vi "Acquire_wp_nodt.vi"(1 "Command FIFO":refnum<k21>, 2 "Circular Buffer Mem":refnum<k21>, 3 "circular buffer length":u32=300, 5 "FPGA I/O In":refnum<k21>="IO Module\\AI A0", 6 "Timing FIFO":refnum<k21>, 7 "channel on/off":bool, 9 "Trigger":i16=1500, 11 "Samples to Acquire":u32=95, 12 "Is Test Pulse?":bool, 13 "# of pretrigger":u32=15, 14 "timing":u64) -> ()   [LabVIEW 2012]
uses:
  <vilib>/rvi/eio/common/nirviEmuTemplateMethod_errors.vi
  <vilib>/rvi/DataTransferAndStorage/Container/Common/niFpgaContainerExecOnDevCompGetState.vi
  <vilib>/rvi/Emulation/niFpgaSctlEmulationGetInTimedLoop.vi
  <vilib>/rvi/DataTransferAndStorage/Container/Common/niFpgaContainerGetUniqueNameForEmu.vi
  <vilib>/rvi/FIFO/Fifo_Resource/nirvififoEmulationSetSize.vi
  <vilib>/rvi/errors/niFpgaSetErrorForExecOnDevCompSimple.vi
  <vilib>/rvi/eio/common/nirviEmuReportErrorAndStop.vi
  <vilib>/rvi/Emulation/niFpgaSctlEmulationFifoFullMgr.vi
  <vilib>/rvi/Emulation/niFpgaSctlEmulationResourceMgr.vi
  <vilib>/rvi/interface/RandomDataEmulation/nirviRandomDataFPGAFIFO.vi
  <vilib>/rvi/interface/RandomDataEmulation/niFpgaRandomDataHandleErrors.vi
  <vilib>/eio/EIONode/EIONode.xnode
  <vilib>/rvi/DataTransferAndStorage/Container/XNode/niFpgaContainer.xnode
  <vilib>/rvi/FIFO/Fifo_Resource/niFpgaFifoEmulationRefIn.vi
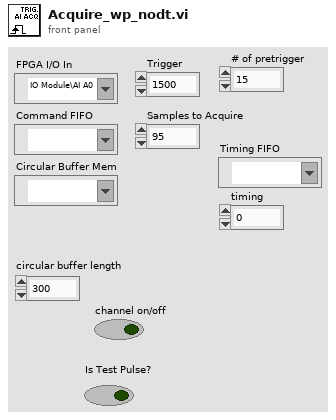
[diagram p1: front panel]
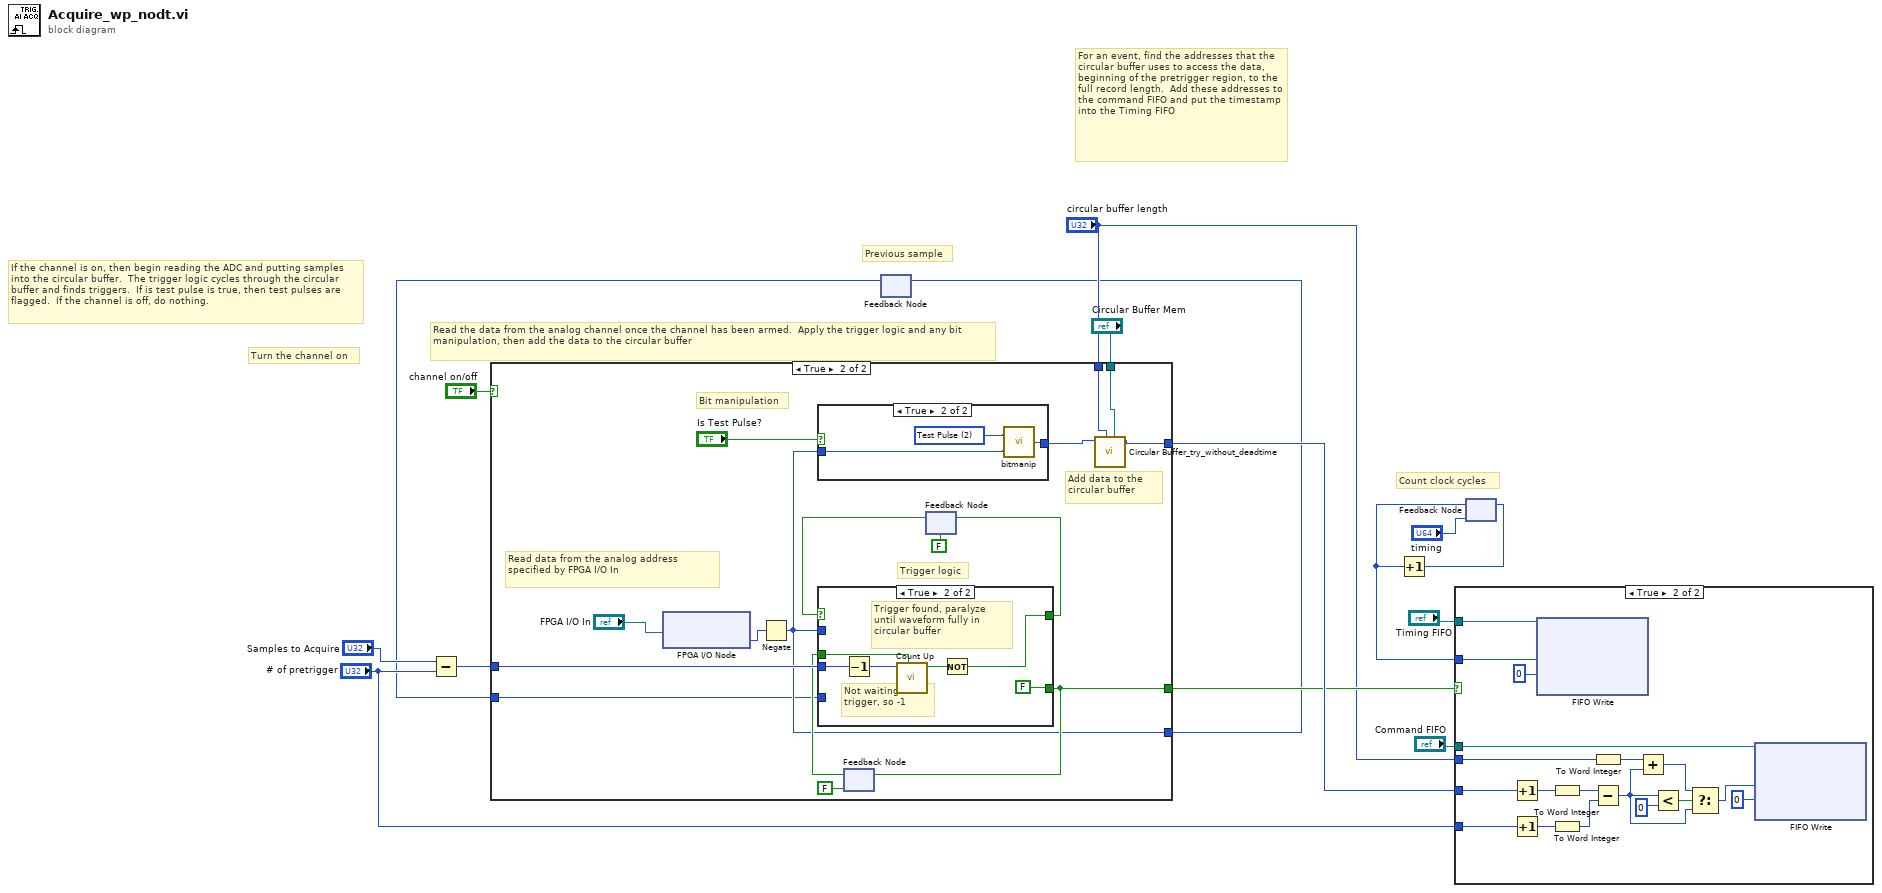
[diagram p0: block diagram]
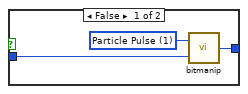
[diagram p4: hidden frame]
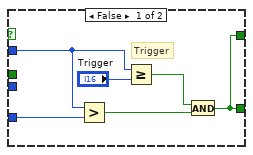
[diagram p5: hidden frame]
diagram:
  # "Previous sample"
  # "Count clock cycles"
  # "For an event, find the addresses that the circular buffer uses to access the data, beginning of the pretrigger region, to the full record length.  Add these addresses to the command FIFO and put the timestamp into the Timing FIFO"
  # "Read the data from the analog channel once the channel has been armed.  Apply the trigger logic and any bit manipulation, then add the data to the circular buffer"
  # "If the channel is on, then begin reading the ADC and putting samples into the circular buffer.  The trigger logic cycles through the circular buffer and finds triggers.  If is test pulse is true, then test pulses are flagged.  If the channel is off, do nothing."
  # "Turn the channel on"
  n1 = Subtract(x="Samples to Acquire", y="# of pretrigger") -> (x-y=w1:u32)
  n2 = feedback #1() -> (w2:i16)  [unwired: 1 in]
  n3 = case shown="True" "channel on/off" {
    tunnel: "Circular Buffer Mem" -> [_ w17]
    tunnel: "circular buffer length" -> [_ w18]
    tunnel: [_ w16] -> w15
    tunnel: w1 -> [_ w29]
    tunnel: [_ w24] -> w14
    tunnel: [_ w23] -> w3
    tunnel: w2 -> [_ w22]
    frame False {
    }
    frame True {
      # "Trigger logic"
      # "Read data from the analog address specified by FPGA I/O In"
      # "Add data to the circular buffer"
      # "Bit manipulation"
      n4 = xnode "FPGA I/O Node"("FPGA I/O In"="FPGA I/O In") -> ("I/O Item"=w20:i16)  [unwired: 1 out]
      n5 = Negate(x=w20) -> (-x=w23:i16)
      n6 = case shown="True" "Is Test Pulse?" {
        tunnel: w23 -> [w33 w36]
        tunnel: [w32 w35] -> w19
        frame False {
          w34 = u16 1 items=["Header Information", "Particle Pulse", "Test Pulse"] ("Pulse Type")
          n7 = call "bitmanip.vi"("Pulse Type"=w34, "Integer to be written"=w33) -> ("Integer Written"=w32:i16)  [unwired: 2 in]
        }
        frame True {
          w37 = u16 2 items=["Header Information", "Particle Pulse", "Test Pulse"] ("Pulse Type")
          n8 = call "bitmanip.vi"("Pulse Type"=w37, "Integer to be written"=w36) -> ("Integer Written"=w35:i16)  [unwired: 2 in]
        }
      }
      n9 = feedback #2(FALSE) -> (w26:bool)
      n10 = feedback #3(FALSE) -> (w28:bool)
      n11 = case shown="True" w28 {
        tunnel: w23 -> [w40 _]
        tunnel: w29 -> [_ w45]
        tunnel: w26 -> [_ w49]
        tunnel: [w42 w47] -> w27
        tunnel: [w42 FALSE] -> w24
        tunnel: w22 -> [w38 _]
        frame False {
          # "Trigger"
          n12 = Greater?(x=w40, y=w38) -> (0:w39:bool)
          n13 = Greater Or Equal?(x=w40, y="Trigger") -> (x >= y?=w41:bool)
          n14 = And(x=w41, y=w39) -> (x .and. y?=w42:bool)
        }
        frame True {
          # "Not waiting for trigger, so -1"
          # "Trigger found, paralyze until waveform fully in circular buffer"
          n15 = Decrement(x=w45) -> (x-1=w44:u32)
          n16 = call "Count Up.vi"("Reset?"=w49, "goal"=w44) -> ("Count Met"=w48:bool)  [unwired: 8 in, 1 out]
          n17 = Not(x=w48) -> (.not. x?=w47:bool)
        }
      }
      n18 = feedback-in #2(w24) -> ()
      n19 = feedback-in #3(w27) -> ()
      n20 = call "Circular Buffer_try_without_deadtime.vi"("Refnum in"=w17, "circular buffer length"=w18, "Data"=w19) -> ("Address"=w16:u16)  [unwired: 8 in]
    }
  }
  n21 = feedback-in #1(w3) -> ()
  n22 = feedback #4("timing") -> (w4:u64)
  n23 = Increment(x=w4) -> (x+1=w5:u64)
  n24 = case shown="True" w14 {
    tunnel: "Command FIFO" -> [_ w67]
    tunnel: "Timing FIFO" -> [_ w66]
    tunnel: w15 -> [_ w55]
    tunnel: "circular buffer length" -> [_ w53]
    tunnel: "# of pretrigger" -> [_ w50]
    tunnel: w4 -> [_ w52]
    frame False {
    }
    frame True {
      n25 = Increment(x=w55) -> (x+1=w61:u16)
      n26 = Increment(x=w50) -> (x+1=w51:u32)
      n27 = xnode ("FIFO Write")("Element"=w52, "Timeout"=0, "FIFO In"=w66) -> ()  [unwired: 2 out]
      n28 = To Word Integer(number=w61) -> (16bit integer=w62:i16)
      n29 = To Word Integer(number=w51) -> (16bit integer=w63:i16)
      n30 = To Word Integer(number=w53) -> (16bit integer=w60:i16)
      n31 = Subtract(x=w62, y=w63) -> (x-y=w59:i16)
      n32 = Add(x=w60, y=w59) -> (x+y=w58:i16)
      n33 = Less?(x=w59, y=i16 0) -> (x < y?=w56:bool)
      n34 = Select(t=w58, s=w56, f=w59) -> (s? t:f=w54:i16)
      n35 = xnode ("FIFO Write")("Element"=w54, "Timeout"=0, "FIFO In"=w67) -> ()  [unwired: 2 out]
    }
  }
  n36 = feedback-in #4(w5) -> ()
